vi "Read Channel Status.vi"(8 "error in (no error)":errorcluster, 11 "Mixer in":refnum<class "Mixer.lvclass">) -> (0 "error out":errorcluster, 2 "Channel Status":T1[](array[typedef]), 3 "Mixer out":refnum<class "Mixer.lvclass">)   [LabVIEW 2020, in "G-Audio.lvlib" / "Mixer.lvclass"]
doc: "Get the status of all mixer channels."
uses:
  Mixer.lvclass
  Channel/Controls/Channel Status.ctl
  Channel/Controls/Channel State.ctl
  Mixer.lvclass/Mixer.ctl
  Channel/Channel.lvclass
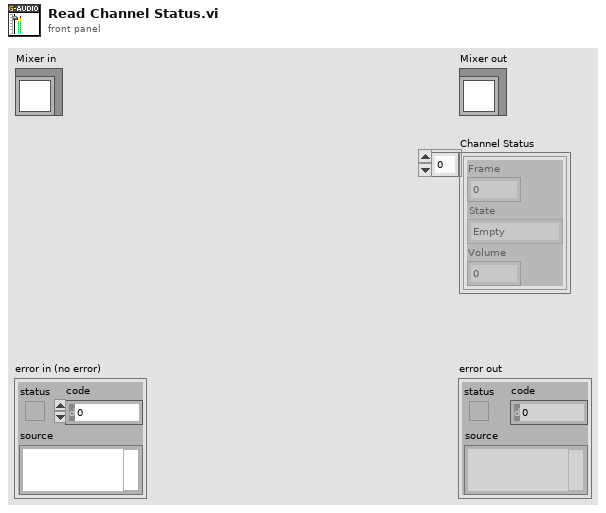
[diagram p1: front panel]
types:
  T1 = typedef "G-Audio.lvlib/Channel.lvclass/Channel Status.ctl" = cluster{"Frame":u64, "State":T2, "Volume":sgl}
  T2 = typedef "G-Audio.lvlib/Channel.lvclass/Channel State.ctl" = enum16{"Empty", "Loading", "Stopped", "Paused", "Playing", "Retrigger"}
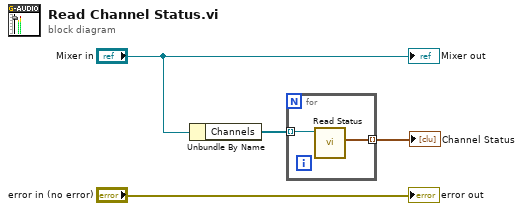
[diagram p0: block diagram]
diagram:
  n1 = Unbundle By Name("Mixer in") -> ("Channels"=w4:refnum<data-value>[])
  n2 = for {
    tunnel: w4 -> [w6] mode=indexing
    tunnel: [w5] -> w1 mode=indexing
    n3 = call "Read Status.vi"("Channel in"=w6) -> ("Channel Status"=w5:T1)  [unwired: 8 in, 2 out]
  }
  "Channel Status" <- w1
  "error out" <- "error in (no error)"
  "Mixer out" <- "Mixer in"
